vi "Auto Select Interface.vi"() -> (3 "Selection":u8)   [LabVIEW 2014]
uses:
  <vilib>/gmath/NI_Gmath.lvlib
panel:
  in  "Value 7":dbl=1.0 format="%#_13g"
  in  "Value 6":dbl=0.85 format="%#_13g"
  in  "Value 5":dbl=0.75 format="%#_13g"
  in  "Value 4":dbl=0.57 format="%#_13g"
  in  "Value 3":dbl=0.42 format="%#_13g"
  in  "Value 2":dbl=0.28 format="%#_13g"
  in  "Value 1":dbl=0.14 format="%#_13g"
  in  "Value 0":dbl format="%#_13g"
  out "error out":errorcluster
  out "Raw Auton Selector Switch Value":dbl(knob)=0.0012585446438982248 scale=-0.1..1.1 scale format="%.1f"
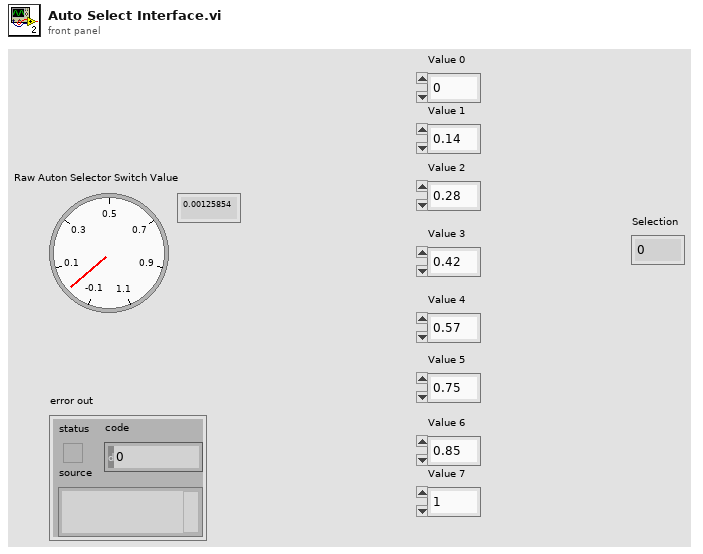
[diagram p1: front panel]
types:
  T1 = typedef "WPI_PotentiometerDevRef.ctl" = cluster{"DevStatus":errorcluster, "Controller":T2, "Analog Channel":T3, "Invert Output":bool}
  T2 = typedef "FPGA_TypedefAnalogModule.ctl" = enum16{"Controller 1"}
  T3 = typedef "FPGA_AIChannel.ctl" = enum8{"AI 0", "AI 1", "AI 2", "AI 3", "AI MXP 0", "AI MXP 1", "AI MXP 2", "AI MXP 3", "Invalid"}
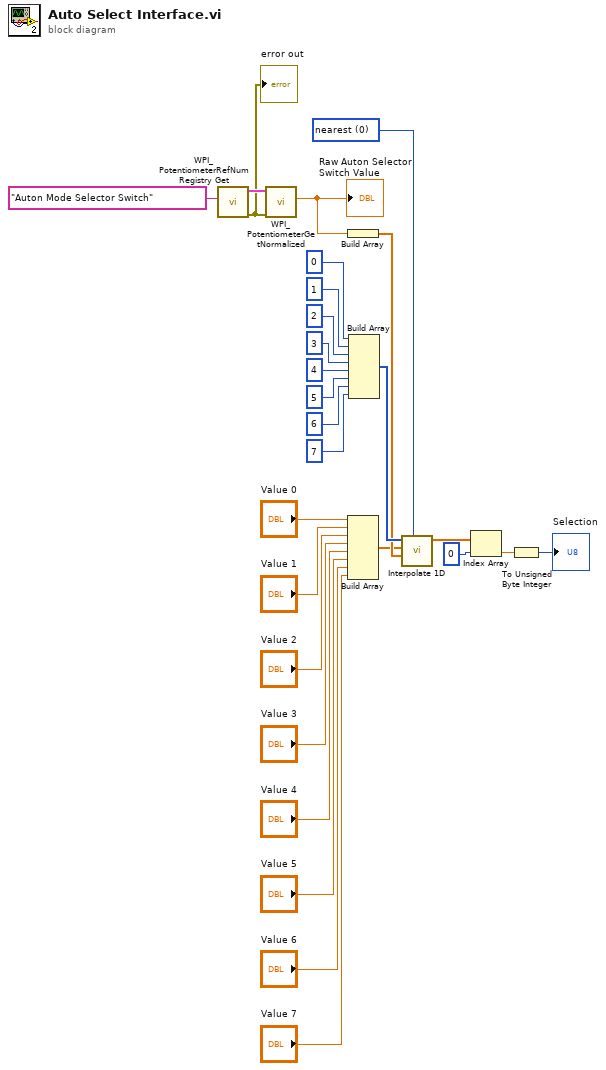
[diagram p0: block diagram]
diagram:
  w7 = 0 items=["nearest", "linear", "spline", "cubic Hermite", "Lagrange"] ("method")
  n1 = call <vilib>:"WPI_PotentiometerRefNum Registry Get.vi"("refnum name"="Auton Mode Selector Switch") -> ("error out"=w26:errorcluster, "PotDevRef"=w27:T1)  [unwired: 9 in]
  "error out" <- w26
  n2 = call <vilib>:"WPI_PotentiometerGetNormalized.vi"("error in"=w26, "PotDevRef"=w27) -> ("Normalized Value"=w2:dbl)  [unwired: 7 in, 2 out]
  "Raw Auton Selector Switch Value" <- w2
  n3 = Build Array(w2) -> (w8:dbl[])
  n4 = Build Array("Value 0", "Value 1", "Value 2", "Value 3", "Value 4", "Value 5", "Value 6", "Value 7") -> (w1:dbl[])
  n5 = Build Array(0, 1 ("element"), 2 ("element"), 3 ("element"), 4 ("element"), 5 ("element"), 6 ("element"), 7 ("element")) -> (w9:i32[])
  n6 = call <vilib>:"Interpolate 1D.vi"("method"=w7, "xi"=w8, "X"=w1, "Y"=w9) -> ("yi"=w6:dbl[])  [unwired: 5 in, 2 out]
  n7 = Index Array(array=w6, index=0) -> (element=w3:dbl)
  n8 = To Unsigned Byte Integer(number=w3) -> (unsigned 8bit integer=→"Selection":u8)
